vi "Rpt _Get _IPQCInspection Testing Data.vi"(0 "Traceability 引用句柄":refnum<k24>, 1 "DateTo":string, 2 "Type":string, 5 "Model":string, 7 "Process":string, 9 "DateFrom":string, 11 "error in (no error)":errorcluster caption="错误输入（无错误）", 12 "ProdID":string) -> (4 "Traceability 引用句柄输出":refnum<k24>, 6 ".NET:System.Data.DataSet":T1={"CaseSensitive"=FALSE, "Container"=refnum, "DataSetName"="", "DefaultViewManager"=refnum, "DesignMode"=FALSE, "EnforceConstraints"=FALSE, "ExtendedProperties"=refnum, "HasErrors"=FALSE, "IsInitialized"=FALSE, "Locale"=refnum, "Namespace"="", "Prefix"="", "Relations"=refnum, "RemotingFormat"=0, "SchemaSerializationMode"=1, "Site"=refnum, "Tables"=refnum} {"SchemaSerializationMode" items=["IncludeSchema"=1, "ExcludeSchema"=2]; "RemotingFormat" items=["Xml", "Binary"]}, 15 "error out":errorcluster caption="错误输出")   [LabVIEW 2014, in "Traceability.lvlib"]
uses:
  D:/webservice/Traceability.dll
  Traceability.dll
  System.Data
  Traceability.lvlib
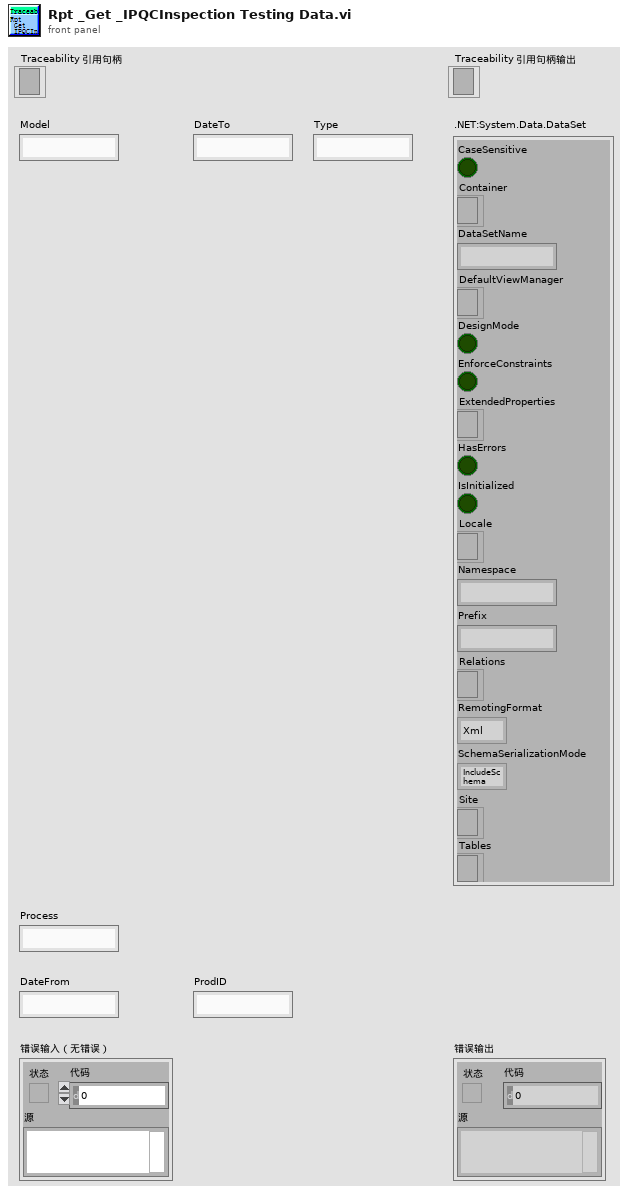
[diagram p1: front panel]
types:
  T1 = cluster{"CaseSensitive":bool, "Container":refnum<k24>, "DataSetName":string, "DefaultViewManager":refnum<k24>, "DesignMode":bool, "EnforceConstraints":bool, "ExtendedProperties":refnum<k24>, "HasErrors":bool, "IsInitialized":bool, "Locale":refnum<k24>, "Namespace":string, "Prefix":string, "Relations":refnum<k24>, "RemotingFormat":i32, "SchemaSerializationMode":i32, "Site":refnum<k24>, "Tables":refnum<k24>}
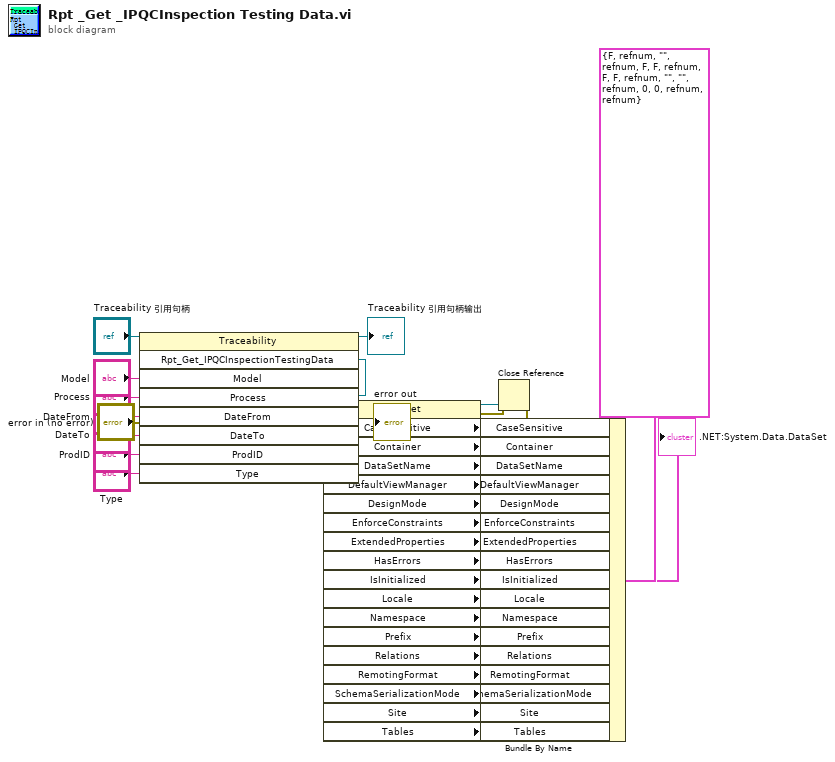
[diagram p0: block diagram]
diagram:
  n1 = invoke class="Traceability" method="Rpt_Get_IPQCInspectionTestingData"(reference="Traceability 引用句柄", error in="error in (no error)", "Model"="Model", "Process"="Process", "DateFrom"="DateFrom", "DateTo"="DateTo", "ProdID"="ProdID", "Type"="Type") -> (reference out=→"Traceability 引用句柄输出":refnum<k24>, error out=w4:errorcluster, "Rpt_Get_IPQCInspectionTestingData"=w30:refnum<k24>)  [unwired: 1 in, 6 out]
  n2 = property class="DataSet"(reference=w30, error in=w4) -> (reference out=w3:refnum<k24>, error out=w2:errorcluster, "CaseSensitive"=w27:bool, "Container"=w26:refnum<k24>, "DataSetName"=w25:string, "DefaultViewManager"=w24:refnum<k24>, "DesignMode"=w23:bool, "EnforceConstraints"=w22:bool, "ExtendedProperties"=w21:refnum<k24>, "HasErrors"=w20:bool, "IsInitialized"=w19:bool, "Locale"=w18:refnum<k24>, "Namespace"=w17:string, "Prefix"=w16:string, "Relations"=w15:refnum<k24>, "RemotingFormat"=w14:i32, "SchemaSerializationMode"=w13:i32, "Site"=w12:refnum<k24>, "Tables"=w11:refnum<k24>)
  n3 = Bundle By Name(cluster=T1 {"CaseSensitive"=FALSE, "Container"=refnum, "DataSetName"="", "DefaultViewManager"=refnum, "DesignMode"=FALSE, "EnforceConstraints"=FALSE, "ExtendedProperties"=refnum, "HasErrors"=FALSE, "IsInitialized"=FALSE, "Locale"=refnum, "Namespace"="", "Prefix"="", "Relations"=refnum, "RemotingFormat"=0, "SchemaSerializationMode"=0, "Site"=refnum, "Tables"=refnum} (".NET:System.Data.DataSet"), "CaseSensitive"=w27, "Container"=w26, "DataSetName"=w25, "DefaultViewManager"=w24, "DesignMode"=w23, "EnforceConstraints"=w22, "ExtendedProperties"=w21, "HasErrors"=w20, "IsInitialized"=w19, "Locale"=w18, "Namespace"=w17, "Prefix"=w16, "Relations"=w15, "RemotingFormat"=w14, "SchemaSerializationMode"=w13, "Site"=w12, "Tables"=w11) -> (→".NET:System.Data.DataSet":T1)
  n4 = Close Reference(reference=w3, error in (no error)=w2) -> (error out=→"error out":errorcluster)
